vi "VI_correctGraphScale.vi"(8 "error in (no error)":errorcluster, 11 "Common Refs in":T1={"LBox_ChList"=refnum, "OXY_SCPI Ref"="TCPIP0::192.168.1.75::10001::SOCKET", "STR_ChName1"=refnum, "STR_ChName2"=refnum, "STR_ChName3"=refnum, "STR_ChName4"=refnum, "STR_ChName5"=refnum, "STR_ChName6"=refnum, "Button_Stop"=refnum, "Button_Start"=refnum, "Button_Disconnect"=refnum, "Button_Connect"=refnum, "Bool_StatusLED"=refnum, "DS Ref"="TCPIP0::192.168.1.75::10001::SOCKET", "Button_SetPort"=refnum, "Button_GetPort"=refnum, "Button_GetState"=refnum, "Button_Reset"=refnum, "Button_Init"=refnum, "STR_UserCMD"=refnum, "STR_CmdPromp"=refnum, "Port"=refnum, "Button_QuerryChs"=refnum, "Graph"=refnum, "STR_ConnAddress"=refnum}) -> (0 "error out":errorcluster)   [LabVIEW 2020]
uses:
  TypeDefs/Refs_Common.ctl
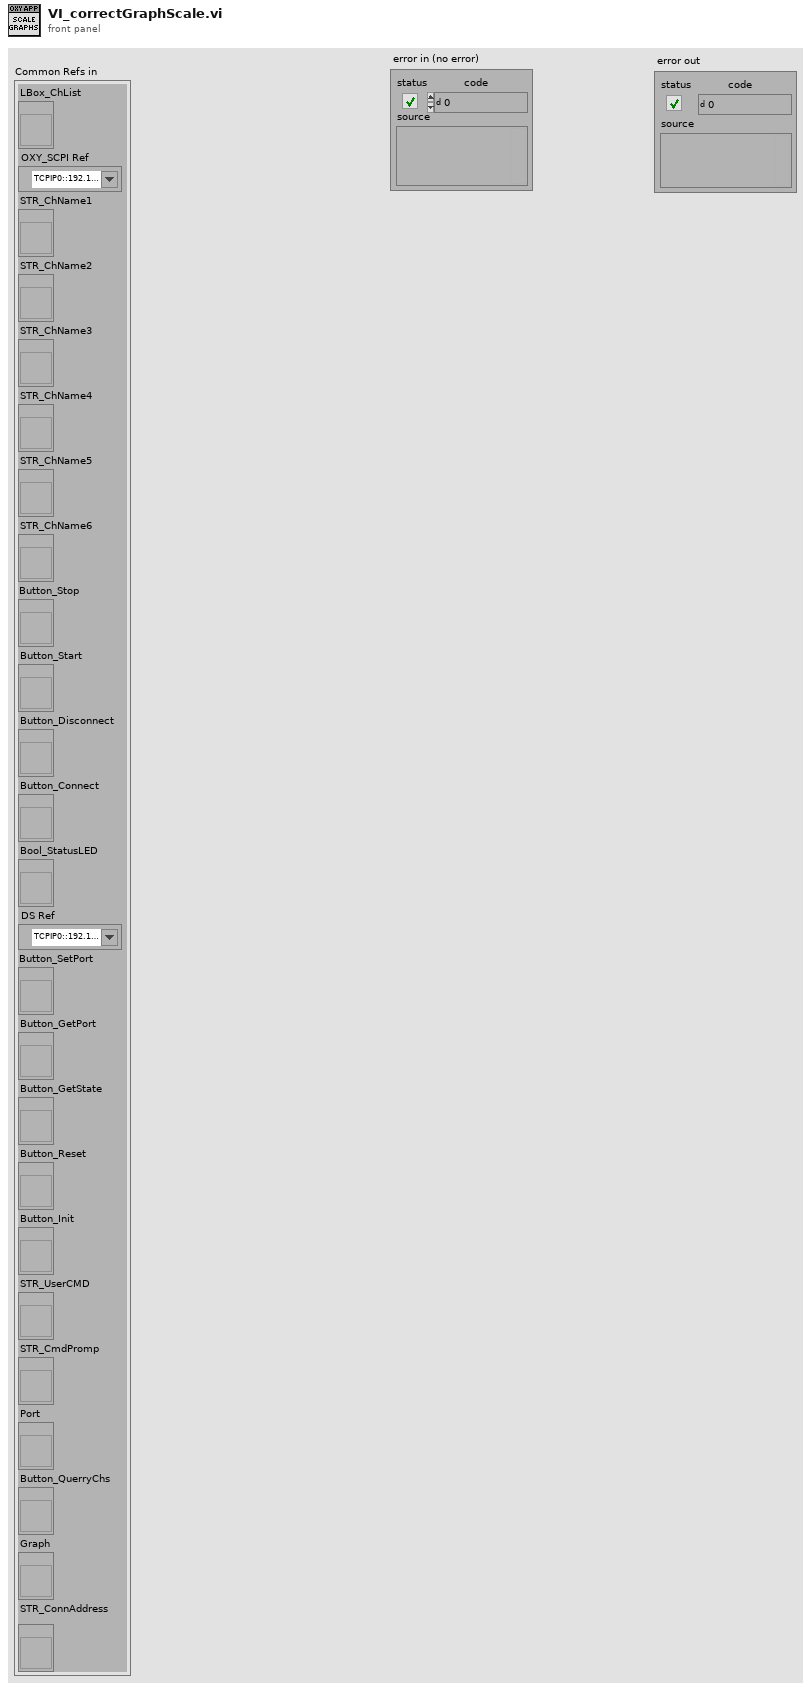
[diagram p1: front panel]
types:
  T1 = typedef "Refs_Common.ctl" = cluster{"LBox_ChList":refnum<vi>, "OXY_SCPI Ref":refnum<visa-resource-name>, "STR_ChName1":refnum<vi>, "STR_ChName2":refnum<vi>, "STR_ChName3":refnum<vi>, "STR_ChName4":refnum<vi>, "STR_ChName5":refnum<vi>, "STR_ChName6":refnum<vi>, "Button_Stop":refnum<vi>, "Button_Start":refnum<vi>, "Button_Disconnect":refnum<vi>, "Button_Connect":refnum<vi>, "Bool_StatusLED":refnum<vi>, "DS Ref":refnum<visa-resource-name>, "Button_SetPort":refnum<vi>, "Button_GetPort":refnum<vi>, "Button_GetState":refnum<vi>, "Button_Reset":refnum<vi>, "Button_Init":refnum<vi>, "STR_UserCMD":refnum<vi>, "STR_CmdPromp":refnum<vi>, "Port":refnum<vi>, "Button_QuerryChs":refnum<vi>, "Graph":refnum<vi>, "STR_ConnAddress":refnum<vi>}
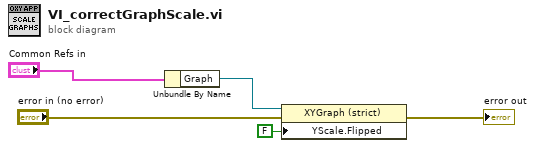
[diagram p0: block diagram]
diagram:
  n1 = Unbundle By Name("Common Refs in") -> ("Graph"=w3:refnum<vi>)
  n2 = property class="XYGraph (strict)"(reference=w3, error in="error in (no error)", "YScale.Flipped"=FALSE ("Y Scale.Flipped")) -> (error out=→"error out":errorcluster)  [unwired: 1 out]
